vi "validPath.vi"(1 "Path":path) -> (15 "Valid?":bool)   [LabVIEW 2017, in "shared.lvlib"]
uses:
  shared.lvlib
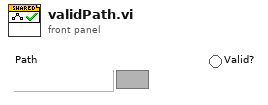
[diagram p1: front panel]
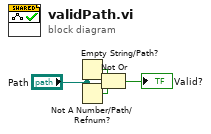
[diagram p0: block diagram]
diagram:
  n1 = Empty String/Path?(string/path="Path") -> (empty?=w3:bool)
  n2 = Not A Number/Path/Refnum?(number/path/refnum="Path") -> (NaN/Path/Refnum?=w4:bool)
  n3 = Not Or(1:w4, 2:w3) -> (0:→"Valid?":bool)
